vi "Autonomous Independent.vi"() -> ()   [LabVIEW 2014]
doc: "This VI is called when autonomous begins, and will automatically be terminated when autonomous ends. You can carry out timed or sensor driven robot movement independently without needing to return to the caller."
uses:
  Lightning base/TeleopCmd.ctl
  Lightning base/CmdFlag.ctl
  Lightning base/Co-Pilot_game_control.ctl
  Lightning base/Auton Modes.ctl
  <vilib>/Rock Robotics/Network Tables/SD Read Number.vi
panel:
  out "Numeric":dbl
  out "error out":errorcluster
  # "Be sure to right-click and choose Data Operations>>Make Current Value default if you want to save the array values with the VI"
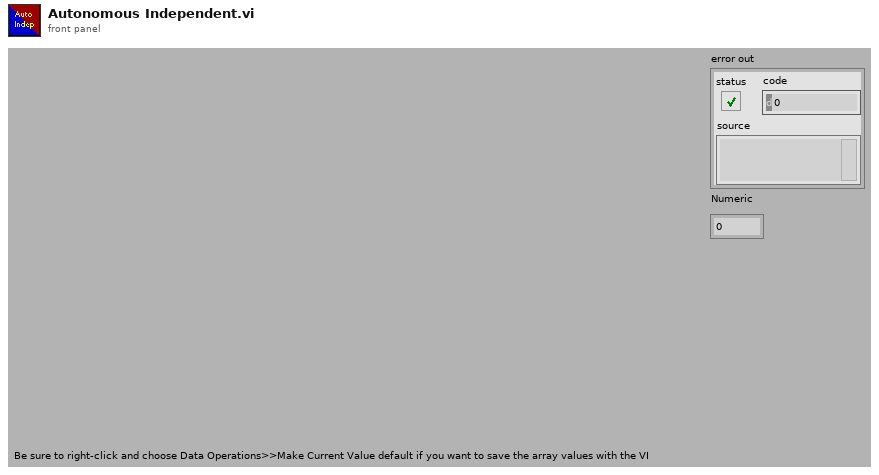
[diagram p1: front panel]
types:
  T1 = typedef "Auton Modes.ctl" = enum16{"Do Nothing", "Snake", "Move Forward", "Move Forward w/Tote", "Move Forward w/RC", "Gather RC from Step", "3 Tote Auton", "Vision Test", "Strafer"}
  T2 = typedef "Co-Pilot_game_control.ctl" = cluster{"Left_Intake":dbl, "Right_Intake":dbl, "Time Stamp":u32, "Command":enum16{"Noop", "Flagged"}, "ToggleCollector":bool, "ManualLift":dbl, "Top_Limit_Switch":bool, "Bottom_Limit_Switch ":bool, "LifterOverride":bool, "AutoLift":i32, "Toggle Auto Lifter":bool, "Activate HP indexer":bool}
  T3 = typedef "TeleopCmd.ctl" = cluster{"CmdFlag":T4, "throttle":dbl, "turn":dbl, "Override":bool, "Strafe":dbl, "MotorPwrMax":u8, "Time":u32, "ultrasonic override":bool}
  T4 = typedef "CmdFlag.ctl" = enum16{"noop", "logflag", "suspend", "resume"}
  T5 = cluster{"proportional gain (Kc)":dbl, "integral time (Ti, min)":dbl, "derivative time (Td, min)":dbl}
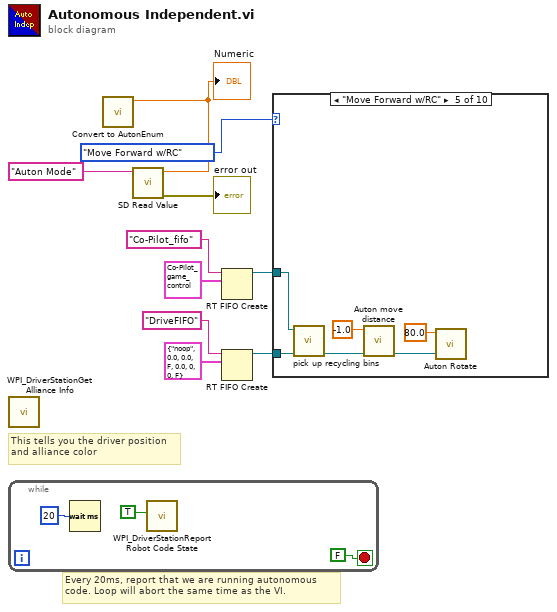
[diagram p0: block diagram]
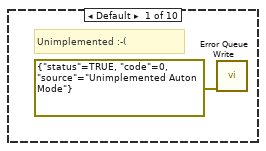
[diagram p2: hidden frame]
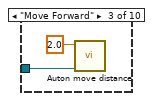
[diagram p4: hidden frame]
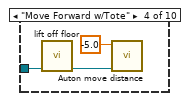
[diagram p5: hidden frame]
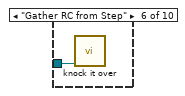
[diagram p6: hidden frame]
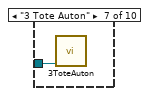
[diagram p7: hidden frame]
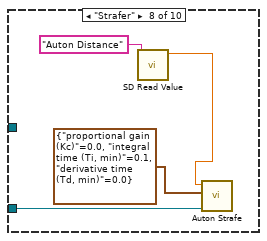
[diagram p8: hidden frame]
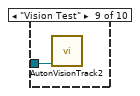
[diagram p9: hidden frame]
diagram:
  # "Every 20ms, report that we are running autonomous\ncode. Loop will abort the same time as the VI."
  # "This tells you the driver position\nand alliance color"
  n1 = call <vilib>:"WPI_DriverStationGet Alliance Info.vi"() -> ()  [unwired: 12 out]
  n2 = while {
    stop <- FALSE stop-if-true
    n3 = Wait (ms)(milliseconds to wait=u32 20) -> ()  [unwired: 1 out]
    n4 = call <vilib>:"WPI_DriverStationReport Robot Code State.vi"("Autonomous"=TRUE) -> ()  [unwired: 10 in, 1 out]
  }
  n5 = call-poly <vilib>:"SD Read Value.vi"("Name"="Auton Mode") -> ("error out"=→"error out":errorcluster, "Numeric"=w5:dbl)  [unwired: 8 in, 1 out]
  "Numeric" <- w5
  n6 = call "Convert to AutonEnum.vi"("Auton In"=w5) -> ()  [unwired: 10 in, 1 out]
  n7 = RT FIFO Create(0:"Co-Pilot_fifo" ("name (unnamed)"), 1:T2 {"Left_Intake"=0.0, "Right_Intake"=0.0, "Time Stamp"=0, "Command"=enum."Noop", "ToggleCollector"=FALSE, "ManualLift"=0.0, "Top_Limit_Switch"=FALSE, "Bottom_Limit_Switch "=FALSE, "LifterOverride"=FALSE, "AutoLift"=0, "Toggle Auto Lifter"=FALSE, "Activate HP indexer"=FALSE}) -> (8:w2:refnum<k33>)  [unwired: 6 in, 2 out]
  n8 = RT FIFO Create(0:"DriveFIFO" ("name (unnamed)"), 1:T3 {"CmdFlag"=enum."noop", "throttle"=0.0, "turn"=0.0, "Override"=FALSE, "Strafe"=0.0, "MotorPwrMax"=0, "Time"=0, "ultrasonic override"=FALSE} ("Cluster")) -> (8:w6:refnum<k33>)  [unwired: 6 in, 2 out]
  n9 = case shown="\"Move Forward w/RC\"" Auton_Modes."Move Forward w/RC" ("Auton Out") {
    tunnel: w6 -> [_ _ w15 w17 w23 w26 w27 w31 w32 _]
    tunnel: w2 -> [_ _ _ _ w22 _ _ _ _ _]
    frame Default {
      # "Unimplemented :-("
      n10 = call "Error Queue Write.vi"("error in (no error)"=errorcluster {"status"=TRUE, "code"=0, "source"="Unimplemented Auton Mode"}) -> ()  [unwired: 11 in]
    }
    frame "Do Nothing" {
      # "It works!!!!"
    }
    frame "Move Forward" {
      n11 = call "Auton move distance.vi"("Distance"=2.0, "Refnum in"=w15) -> ()  [unwired: 7 in, 2 out]
    }
    frame "Move Forward w/Tote" {
      n12 = call "lift off floor.vi"("rt fifo in"=w17) -> ("rt fifo out"=w19:refnum<k33>)  [unwired: 9 in]
      n13 = call "Auton move distance.vi"("Distance"=-5.0, "Refnum in"=w19) -> ()  [unwired: 7 in, 2 out]
    }
    frame "Move Forward w/RC" {
      n14 = call "pick up recycling bins.vi"("CoPilot"=w22, "Refnum in"=w23) -> ("Refnum out"=w24:refnum<k33>)  [unwired: 8 in]
      n15 = call "Auton move distance.vi"("Distance"=-1.0, "Refnum in"=w24) -> ("rt fifo out"=w21:refnum<k33>)  [unwired: 7 in, 1 out]
      n16 = call "Auton Rotate.vi"("Rotation"=80.0, "Refnum in"=w21) -> ()  [unwired: 7 in, 2 out]
    }
    frame "Gather RC from Step" {
      n17 = call "knock it over.vi"("Refnum in"=w26) -> ()  [unwired: 10 in, 1 out]
    }
    frame "3 Tote Auton" {
      n18 = call "3ToteAuton.vi"("Refnum in"=w27) -> ()  [unwired: 10 in, 1 out]
    }
    frame "Strafer" {
      n19 = call-poly <vilib>:"SD Read Value.vi"("Name"="Auton Distance") -> ("Numeric"=w29:dbl)  [unwired: 8 in, 2 out]
      n20 = call "Auton Strafe.vi"("Distance"=w29, "PID gains"=T5 {"proportional gain (Kc)"=0.0, "integral time (Ti, min)"=0.1, "derivative time (Td, min)"=0.0}, "Refnum in"=w31) -> ()  [unwired: 6 in, 2 out]
    }
    frame "Vision Test" {
      n21 = call "AutonVisionTrack2.vi"("Refnum in"=w32) -> ()  [unwired: 9 in, 1 out]
    }
    frame "Snake" {
    }
  }
